vi "Ex7_Feu_Signialisation_Var_1.vi"() -> ()   [LabVIEW 2018]
panel:
  in  "Phase 4":u64
  in  "Phase 3":u64
  in  "Phase 2":u64
  in  "Phase":u64
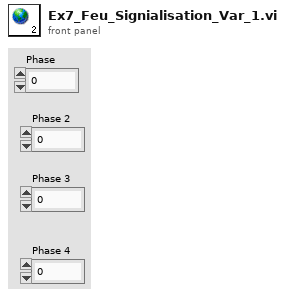
[diagram p1: front panel]
diagram:
